vi "Get Module Info.vi"(8 "error in (no error)":errorcluster) -> (0 "error out":errorcluster, 1 "Execution State":T1(ring), 2 "isModuleRunning?":bool, 3 "Module Ref":refnum<vi>)   [LabVIEW 2014, in "Chart Module.lvlib"]
uses:
  Chart Module.lvlib
  Main.vi
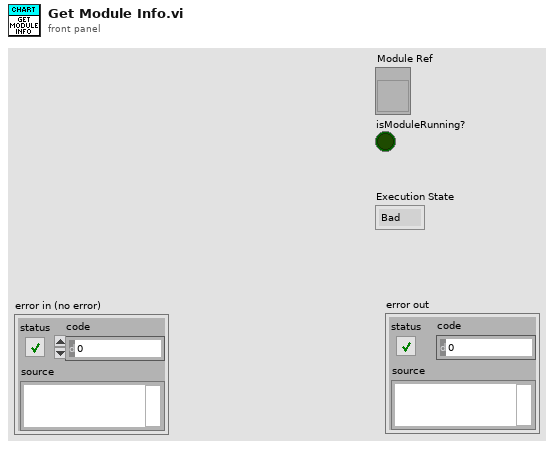
[diagram p1: front panel]
types:
  T1 = enum32{"Bad", "Idle", "Run top level", "Running"}
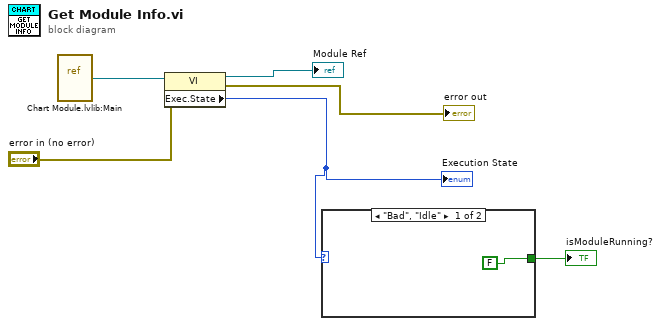
[diagram p0: block diagram]
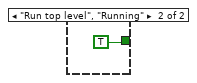
[diagram p2: hidden frame]
diagram:
  n1 = vi-ref "Chart Module.lvlib:Main.vi"() -> (w6:refnum<vi>)
  n2 = property class="VI"(reference=w6, error in="error in (no error)") -> (reference out=→"Module Ref":refnum<vi>, error out=→"error out":errorcluster, "Exec.State"=w2:T1)
  "Execution State" <- w2
  n3 = case shown="\"Bad\", \"Idle\"" w2 {
    tunnel: [FALSE TRUE] -> w1
    frame "Bad", "Idle" {
    }
    frame "Run top level", "Running" {
    }
  }
  "isModuleRunning?" <- w1
